vi "RTS Open All TDMS Files.vi"(8 "error in (no error)":errorcluster, 11 "TDMS Data Save Input":T1) -> (0 "error out":errorcluster, 3 "TDMS Data Save Output":T1)   [LabVIEW 2016]
uses:
  Type Definitions/RTS TDMS Filename Locations.ctl
  Type Definitions/RTS Save References.ctl
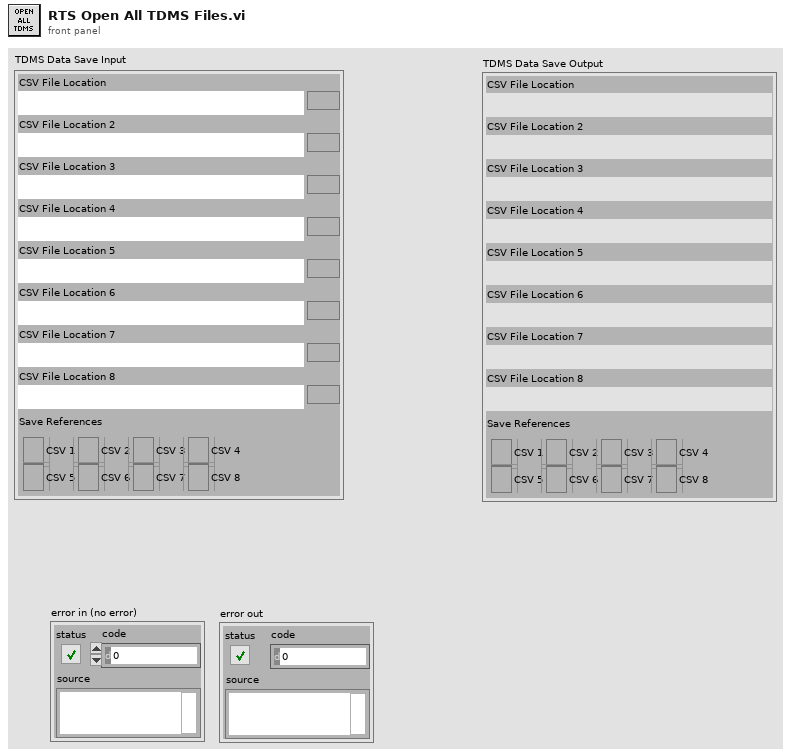
[diagram p1: front panel]
types:
  T1 = typedef "RTS TDMS Filename Locations.ctl" = cluster{"CSV File Location":path, "CSV File Location 2":path, "CSV File Location 3":path, "CSV File Location 4":path, "CSV File Location 5":path, "CSV File Location 6":path, "CSV File Location 7":path, "CSV File Location 8":path, "Save References":T2}
  T2 = typedef "RTS Save References.ctl" = cluster{"CSV 1":refnum<file>, "CSV 2":refnum<file>, "CSV 3":refnum<file>, "CSV 4":refnum<file>, "CSV 5":refnum<file>, "CSV 6":refnum<file>, "CSV 7":refnum<file>, "CSV 8":refnum<file>}
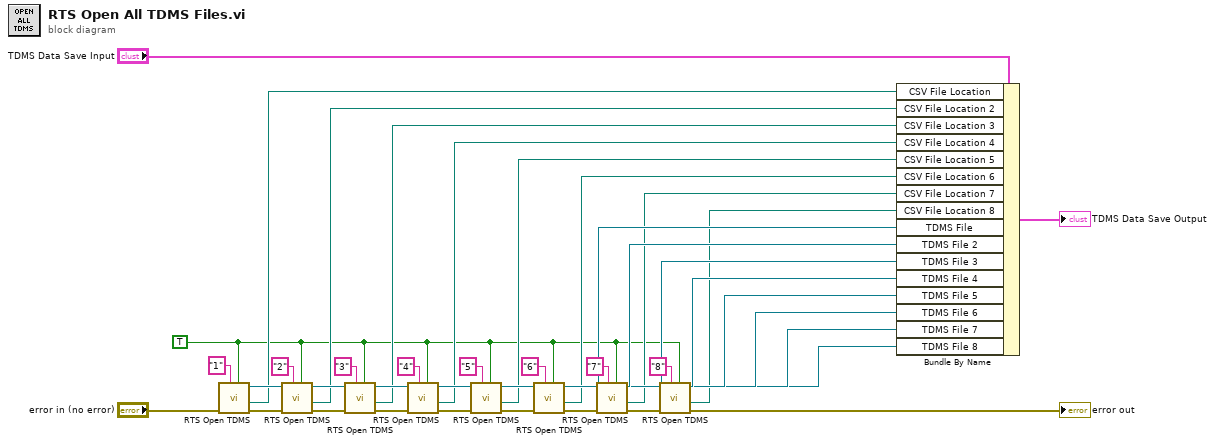
[diagram p0: block diagram]
diagram:
  w1 = TRUE ("Specific File Location?")
  n1 = call "RTS Open TDMS.vi"("Specific File Location?"=w1, "Chamber Number"="1", "error in (no error)"="error in (no error)") -> ("Error Out"=w35:errorcluster, "TDMS File Location"=w30:path, "TDMS File"=w31:refnum<k34>)  [unwired: 5 in, 1 out]
  n2 = call "RTS Open TDMS.vi"("Specific File Location?"=w1, "Chamber Number"="2", "error in (no error)"=w35) -> ("Error Out"=w10:errorcluster, "TDMS File Location"=w28:path, "TDMS File"=w29:refnum<k34>)  [unwired: 5 in, 1 out]
  n3 = call "RTS Open TDMS.vi"("Specific File Location?"=w1, "Chamber Number"="3", "error in (no error)"=w10) -> ("Error Out"=w11:errorcluster, "TDMS File Location"=w26:path, "TDMS File"=w27:refnum<k34>)  [unwired: 5 in, 1 out]
  n4 = call "RTS Open TDMS.vi"("Specific File Location?"=w1, "Chamber Number"="4", "error in (no error)"=w11) -> ("Error Out"=w12:errorcluster, "TDMS File Location"=w25:path, "TDMS File"=w24:refnum<k34>)  [unwired: 5 in, 1 out]
  n5 = call "RTS Open TDMS.vi"("Specific File Location?"=w1, "Chamber Number"="5", "error in (no error)"=w12) -> ("Error Out"=w13:errorcluster, "TDMS File Location"=w23:path, "TDMS File"=w22:refnum<k34>)  [unwired: 5 in, 1 out]
  n6 = call "RTS Open TDMS.vi"("Specific File Location?"=w1, "Chamber Number"="6", "error in (no error)"=w13) -> ("Error Out"=w14:errorcluster, "TDMS File Location"=w20:path, "TDMS File"=w21:refnum<k34>)  [unwired: 5 in, 1 out]
  n7 = call "RTS Open TDMS.vi"("Specific File Location?"=w1, "Chamber Number"="7", "error in (no error)"=w14) -> ("Error Out"=w9:errorcluster, "TDMS File Location"=w18:path, "TDMS File"=w19:refnum<k34>)  [unwired: 5 in, 1 out]
  n8 = call "RTS Open TDMS.vi"("Specific File Location?"=w1, "Chamber Number"="8", "error in (no error)"=w9) -> ("Error Out"=→"error out":errorcluster, "TDMS File Location"=w17:path, "TDMS File"=w16:refnum<k34>)  [unwired: 5 in, 1 out]
  n9 = Bundle By Name(cluster="TDMS Data Save Input", "CSV File Location"=w30, "CSV File Location 2"=w28, "CSV File Location 3"=w26, "CSV File Location 4"=w25, "CSV File Location 5"=w23, "CSV File Location 6"=w20, "CSV File Location 7"=w18, "CSV File Location 8"=w17, "TDMS File"=w31, "TDMS File 2"=w29, "TDMS File 3"=w27, "TDMS File 4"=w24, "TDMS File 5"=w22, "TDMS File 6"=w21, "TDMS File 7"=w19, "TDMS File 8"=w16) -> (→"TDMS Data Save Output":T1)
